vi "generation_TC_modulation.vi"(11 "Numeric":i32) -> (1 "output bit stream":i8[](array[numeric]), 2 "matched filter coefficients":dbl[](array[numeric]), 3 "output complex waveform":T1 {"Y" format="%.3f"; "dt" format="%^.2e"; "t0" format="%.4f"})   [LabVIEW 2018]
uses:
  <vilib>/addons/Modulation/Analog/controls/Complex Data Waveform.ctl
  <vilib>/addons/Modulation/Analog/support/mod_Set Error Source.vi
  <vilib>/addons/Modulation/Digital/Support/Common/Validators/mod_Generate Filter Coefficients Validate.vi
  <vilib>/addons/Modulation/Digital/General/subVIs/mod_Generate Filter Coefficients.vi
  <vilib>/addons/Modulation/Digital/General/MT Generate PSK System Parameters(M).vi
  <vilib>/addons/Modulation/niDMT.lvlib
  <vilib>/addons/Modulation/niAMT.lvlib
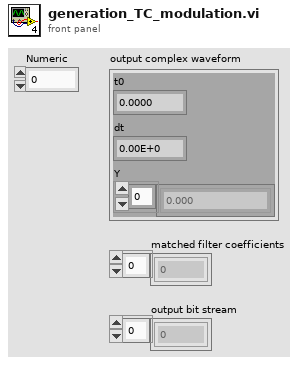
[diagram p1: front panel]
types:
  T1 = typedef "niAMT.lvlib/Complex Data Waveform.ctl" = cluster{"t0":dbl, "dt":dbl, "Y":cdb[]}
  T2 = enum16{"none", "Raised Cosine", "Root Raised Cos", "Gaussian"}
  T3 = cluster{"samples per symbol (16)":i32, "symbol map":cdb[], "differential PSK":enum16{"disable", "enable"}, "PSK type":u16}
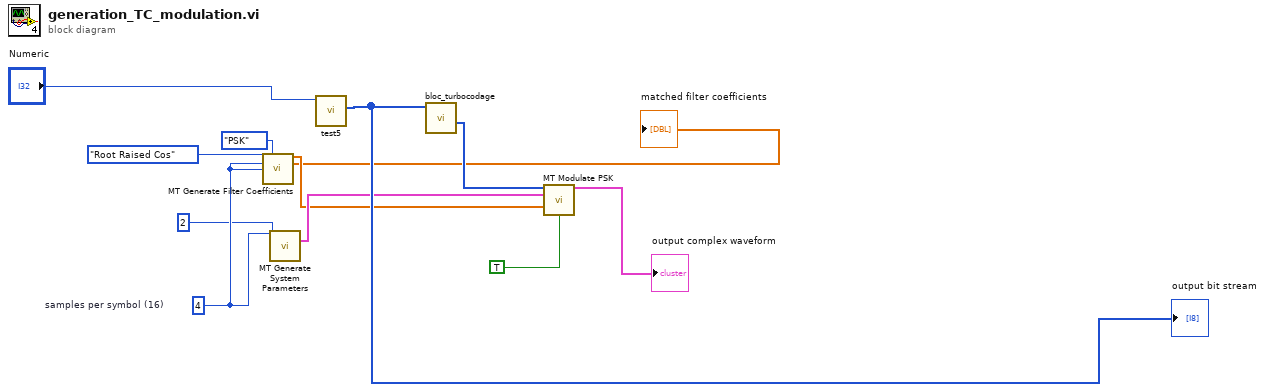
[diagram p0: block diagram]
diagram:
  w12 = 4  # samples per symbol (16)
  n1 = call <vilib>:"MT Generate Filter Coefficients.vi"("pulse shaping filter (none)"=T2."Root Raised Cos", "modulation type"=enum16{"FSK", "PSK", "QAM", "MSK", "PAM", "ASK"}."PSK", "pulse shaping samples per symbol (16)"=w12, "matched samples per symbol (16)"=w12) -> ("pulse shaping filter coefficients"=w3:dbl[], "matched filter coefficients"=→"matched filter coefficients":dbl[])  [unwired: 9 in, 1 out]
  n2 = call-poly <vilib>:"MT Generate System Parameters.vi"("samples per symbol (16)"=w12, "M-PSK (4)"=2) -> ("PSK system parameters"=w5:T3)  [unwired: 11 in, 2 out]
  n3 = call "test5.vi"("k"="Numeric") -> ("output bit stream"=w10:i8[])  [unwired: 9 in, 1 out]
  "output bit stream" <- w10
  n4 = call "bloc_turbocodage.vi"("Array in"=w10) -> ("output bit stream"=w4:i8[])  [unwired: 8 in, 2 out]
  n5 = call <vilib>:"MT Modulate PSK.vi"("input bit stream"=w4, "PSK system parameters"=w5, "pulse shaping filter coefficients"=w3, "reset? (T)"=TRUE) -> ("output complex waveform"=→"output complex waveform":T1)  [unwired: 9 in, 2 out]
